vi "autochange_display.vi"(9 "display ref":refnum<vi>, 10 "delay":u32=3000 caption="delay (3000)", 11 "new val":T1 caption="new part") -> ()   [LabVIEW 2010, in "password.xctl"]
uses:
  password.xctl
  controls/Data.ctl
  delayed_replace_star.vi
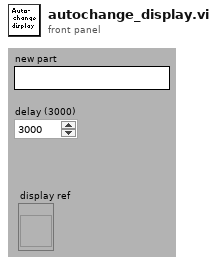
[diagram p1: front panel]
types:
  T1 = typedef "password.xctl/Data.ctl" = string
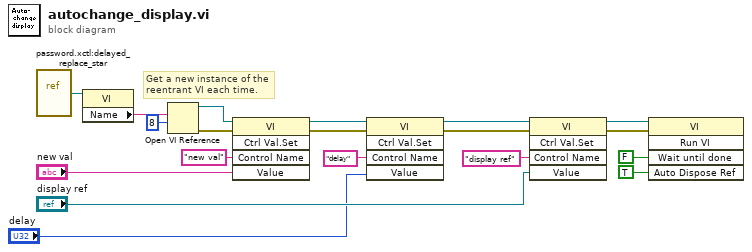
[diagram p0: block diagram]
diagram:
  # "Get a new instance of the \nreentrant VI each time."
  n1 = vi-ref "password.xctl:delayed_replace_star.vi"() -> (w15:refnum<vi>)
  n2 = property class="VI"(reference=w15) -> ("Name"=w14:string)  [unwired: 1 in, 2 out]
  n3 = Open VI Reference(vi path=w14, options=8) -> (vi reference=w9:refnum<vi>, error out=w10:errorcluster)  [unwired: 4 in]
  n4 = invoke class="VI" method="Ctrl Val.Set"(reference=w9, error in=w10, "Control Name"="new val", "Value"="new val") -> (reference out=w6:refnum<vi>, error out=w3:errorcluster)  [unwired: 1 in, 3 out]
  n5 = invoke class="VI" method="Ctrl Val.Set"(reference=w6, error in=w3, "Control Name"="delay", "Value"="delay") -> (reference out=w5:refnum<vi>, error out=w4:errorcluster)  [unwired: 1 in, 3 out]
  n6 = invoke class="VI" method="Ctrl Val.Set"(reference=w5, error in=w4, "Control Name"="display ref", "Value"="display ref") -> (reference out=w12:refnum<vi>, error out=w11:errorcluster)  [unwired: 1 in, 3 out]
  n7 = invoke class="VI" method="Run VI"(reference=w12, error in=w11, "Wait until done"=FALSE ("Wait Until Done"), "Auto Dispose Ref"=TRUE ("Auto Dispose Reference")) -> ()  [unwired: 1 in, 5 out]
